vi "GetGraphTypeInfo.vi"(0 "reference in":refnum<class "ClassDiagramGraph.lvclass">, 5 "error in (no error)":errorcluster) -> (14 "reference out":refnum<class "ClassDiagramGraph.lvclass">, 15 "GraphTypeName":string, 16 "NodeTypes":refnum<class "AbstractNode.lvclass">[](array[class]), 17 "EdgeTypes":refnum<class "AbstractEdge.lvclass">[](array[class]), 18 "GraphTypeUserName":string, 19 "error out":errorcluster)   [LabVIEW 2020, in "ClassDiagramGraph.lvclass"]
uses:
  <resource>/Framework/Providers/Open_GDS/UML/ClassDiagramGraph_class/ClassDiagramGraph.lvclass
  <resource>/Framework/Providers/Open_GDS/UML/AbstractNode_class/AbstractNode.lvclass
  <resource>/Framework/Providers/Open_GDS/UML/AbstractEdge_class/AbstractEdge.lvclass
  <resource>/Framework/Providers/Open_GDS/UML/ClassNode_class/ClassNode.lvclass
  C:/Program Files (x86)/National Instruments/LabVIEW 2020/resource/Framework/Providers/Open_GDS/UML/AbstractNode_class/AbstractNode.lvclass
  <resource>/Framework/Providers/Open_GDS/UML/NoteNode_class/NoteNode.lvclass
  <resource>/Framework/Providers/Open_GDS/UML/PackageNode_class/PackageNode.lvclass
  <resource>/Framework/Providers/Open_GDS/UML/InterfaceNode_class/InterfaceNode.lvclass
  <resource>/Framework/Providers/Open_GDS/UML/ClassRelationshipEdge_class/ClassRelationshipEdge.lvclass
  C:/Program Files (x86)/National Instruments/LabVIEW 2020/resource/Framework/Providers/Open_GDS/UML/GeneralPathEdge_class/GeneralPathEdge.lvclass
  <resource>/Framework/Providers/Open_GDS/UML/NoteEdge_class/NoteEdge.lvclass
  <resource>/Framework/Providers/Open_GDS/UML/PointNode_class/PointNode.lvclass
  <resource>/Framework/Providers/Open_GDS/UML/GeneralPathEdge_class/GeneralPathEdge.lvclass
  C:/Program Files (x86)/National Instruments/LabVIEW 2020/resource/Framework/Providers/Open_GDS/UML/AbstractEdge_class/AbstractEdge.lvclass
  <resource>/Framework/Providers/Open_GDS/UML/Graph_class/Graph.lvclass
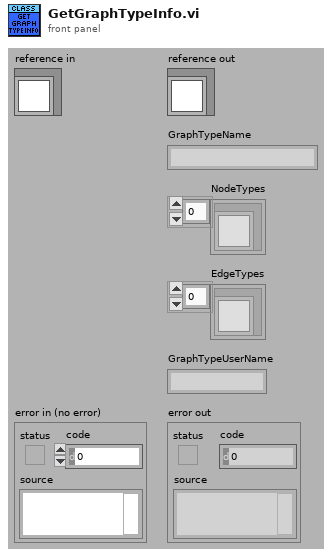
[diagram p1: front panel]
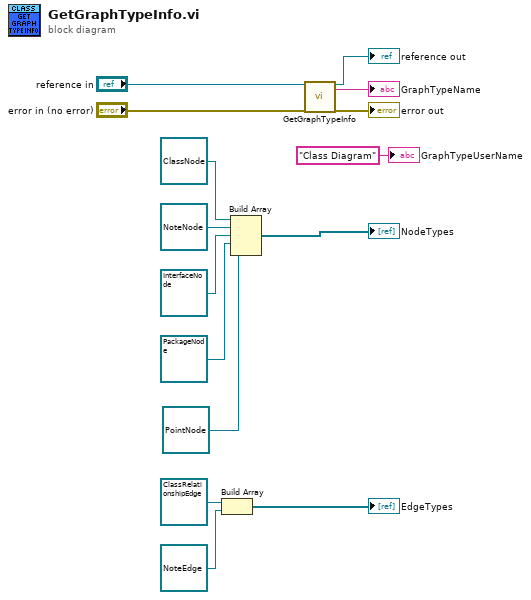
[diagram p0: block diagram]
diagram:
  n1 = Build Array(refnum<class "ClassRelationshipEdge.lvclass"> refnum ("ClassRelationshipEdge.lvclass"), refnum<class "NoteEdge.lvclass"> refnum ("NoteEdge.lvclass")) -> (→"EdgeTypes":refnum<class "GeneralPathEdge.lvclass">[])
  n2 = Build Array(refnum<class "ClassNode.lvclass"> refnum ("ClassNode.lvclass"), refnum<class "NoteNode.lvclass"> refnum ("NoteNode.lvclass"), refnum<class "InterfaceNode.lvclass"> refnum ("InterfaceNode.lvclass"), refnum<class "PackageNode.lvclass"> refnum ("PackageNode.lvclass"), refnum<class "PointNode.lvclass"> refnum ("PointNode.lvclass")) -> (→"NodeTypes":refnum<class "AbstractNode.lvclass">[])
  n3 = call-parent "GetGraphTypeInfo.vi"("reference in"="reference in", "error in (no error)"="error in (no error)") -> ("reference out"=→"reference out":refnum<class "ClassDiagramGraph.lvclass">, "GraphTypeName"=→"GraphTypeName":string, "error out"=→"error out":errorcluster)  [unwired: 12 in, 3 out]
  "GraphTypeUserName" <- "Class Diagram" ("GraphTypeUserName")
